vi "Deliver Results.vi"(8 "error in (no error)":errorcluster, 11 "Response Synchronizer in":refnum<class "Response Synchronizer.lvclass">) -> (0 "error out":errorcluster, 2 "Results":refnum<class "Acquired Result.lvclass">[](array[class]), 3 "Response Synchronizer out":refnum<class "Response Synchronizer.lvclass">)   [LabVIEW 2021, in "Response Synchronizer.lvclass"]
uses:
  Response Synchronizer.lvclass
  NHMFL_Core/Libraries/Instruments/Results/Acquired Result/Acquired Result.lvclass
  Response Synchronizer.lvclass/Response Synchronizer.ctl
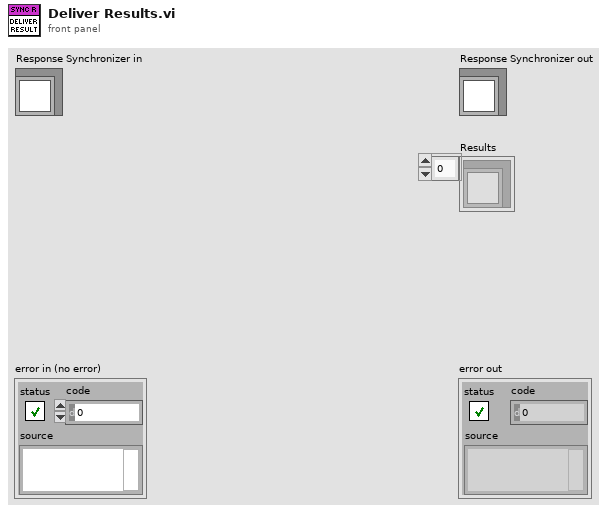
[diagram p1: front panel]
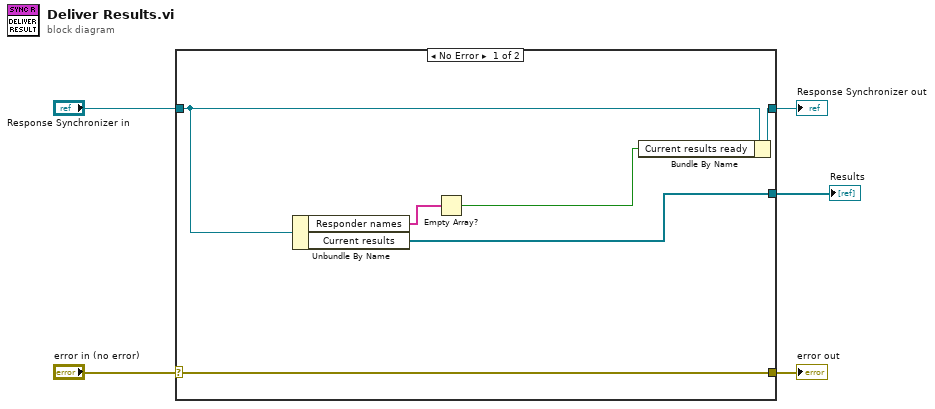
[diagram p0: block diagram]
diagram:
  n1 = case shown="No Error" "error in (no error)" {
    selector: "error in (no error)" -> [w11 w13]
    tunnel: [w11 w13] -> w4
    tunnel: [w8 w12] -> w2
    tunnel: "Response Synchronizer in" -> [w10 w12]
    tunnel: [w9 _] -> w1
    frame No Error {
      n2 = Unbundle By Name(w10) -> ("Responder names"=w7:string[], "Current results"=w9:refnum<class "Acquired Result.lvclass">[])
      n3 = Empty Array?(array=w7) -> (empty?=w6:bool)
      n4 = Bundle By Name(cluster=w10, "Current results ready"=w6) -> (w8:refnum<class "Response Synchronizer.lvclass">)
    }
    frame Error {
    }
  }
  "error out" <- w4
  "Response Synchronizer out" <- w2
  "Results" <- w1
